vi "FPGA testbench.vi"() -> ()   [LabVIEW 2016]
uses:
  <vilib>/rvi/DesktopExecutionNode/Execution/niFpgaDEN_Execute.vi
  <vilib>/rvi/DesktopExecutionNode/DesktopExecutionNode.xnode
panel:
  out "LEDb":bool
  out "LEDa":bool
  out "paused":bool
  in  "pause":bool
  in  "Stop Button":bool
  out "LED 0:3":bool[](array[boolean])
  in  "button":bool
  in  "loop time [ms]":u32
  # "FPGA testbench"
  # "onboard devices"
  # "front-panel controls and indicators"
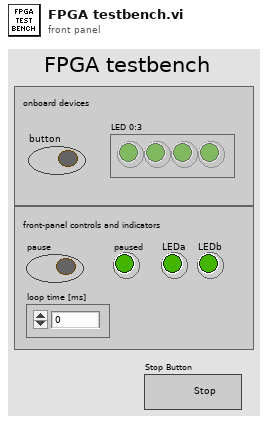
[diagram p1: front panel]
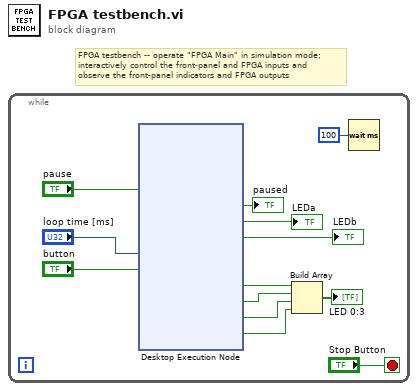
[diagram p0: block diagram]
diagram:
  # "FPGA testbench -- operate \"FPGA Main\" in simulation mode;\ninteractively control the front-panel and FPGA inputs and\nobserve the front-panel indicators and FPGA outputs"
  n1 = while {
    stop <- "Stop Button" stop-if-true
    n2 = xnode "Desktop Execution Node"("pause"="pause", "milliseconds to wait"="loop time [ms]", "Button0"="button") -> ("paused"=→"paused":bool, "LED2"=→"LEDa":bool, "LED3"=→"LEDb":bool, "LED0"=w11:bool, "LED1"=w10:bool, "LED2"=w9:bool, "LED3"=w8:bool)  [unwired: 1 in, 1 out]
    n3 = Build Array(w11, w10, w9, w8) -> (→"LED 0:3":bool[])
    n4 = Wait (ms)(milliseconds to wait=u32 100) -> ()  [unwired: 1 out]
  }
